vi "PWM Coerce Frequency.vi"(10 "Frequency":dbl, 11 "Frequency Units":enum16{"Hz", "kHz"}(ring)) -> (2 "Coerced Frequency":dbl, 3 "Coercion needed?":bool)   [LabVIEW 2021]
uses:
  <vilib>/myRIO/Common/Instrument Driver Framework/Utilities/vis/Calculate Clock Settings.vi
  <vilib>/myRIO/Common/Instrument Driver Framework/Utilities/vis/Calculate TOP (Phase Correct Mode).vi
  <vilib>/myRIO/Common/Instrument Driver Framework/Utilities/vis/Calculate TOP (Normal Mode).vi
  <vilib>/myRIO/Common/Instrument Driver Framework/Utilities/vis/Calculate Frequency (Phase Correct Mode).vi
  <vilib>/myRIO/Common/Instrument Driver Framework/Utilities/vis/Calculate Frequency (Normal Mode).vi
  <vilib>/Utility/error.llb/Error Cluster From Error Code.vi
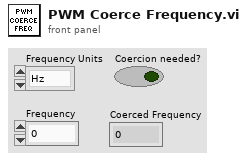
[diagram p1: front panel]
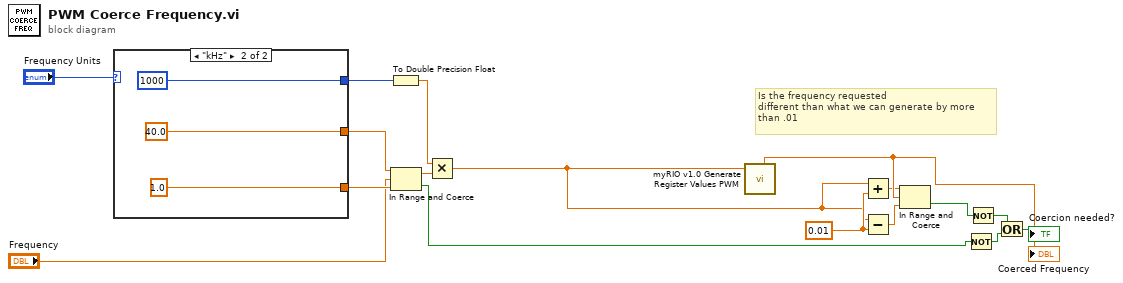
[diagram p0: block diagram]
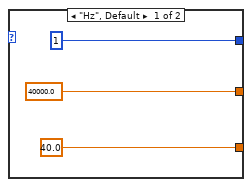
[diagram p2: hidden frame]
diagram:
  w9 = 0.01 ("y")
  # "Is the frequency requested\ndifferent than what we can generate by more\nthan .01"
  n1 = case shown="\"kHz\"" "Frequency Units" {
    tunnel: [1 1000] -> w2
    tunnel: [40000.0 ("Data Entry Limits:Maximum") 40.0 ("Data Entry Limits:Maximum")] -> w5
    tunnel: [40.0 ("Data Entry Limits:Minimum") 1.0 ("Data Entry Limits:Minimum")] -> w17
    frame "Hz", Default {
    }
    frame "kHz" {
    }
  }
  n2 = To Double Precision Float(number=w2) -> (double precision float=w3:dbl)
  n3 = In Range and Coerce(upper limit=w5, x="Frequency", lower limit=w17) -> (coerced(x)=w6:dbl, In Range?=w16:bool)
  n4 = Multiply(x=w3, y=w6) -> (x*y=w1:dbl)
  n5 = call <vilib>:"myRIO v1.0 Generate Register Values PWM.vi"("Frequency (Hz)"=w1) -> ("Actual Frequency (Hz)"=w11:dbl)  [unwired: 6 in, 4 out]
  "Coerced Frequency" <- w11
  n6 = Add(x=w1, y=w9) -> (x+y=w7:dbl)
  n7 = Subtract(x=w1, y=w9) -> (x-y=w8:dbl)
  n8 = In Range and Coerce(upper limit=w7, x=w11, lower limit=w8) -> (In Range?=w12:bool)  [unwired: 1 out]
  n9 = Not(x=w16) -> (.not. x?=w15:bool)
  n10 = Not(x=w12) -> (.not. x?=w13:bool)
  n11 = Or(x=w13, y=w15) -> (x .or. y?=→"Coercion needed?":bool)
